vi "ValueAsDouble.vi"(8 "error in (no error)":errorcluster, 11 "Parameter":string="  <value><double>-12.3456</double></value>\n    ") -> (0 "error out":errorcluster, 3 "value":dbl)   [LabVIEW 2009]
doc: "Convert XML-RPC double to LV double"
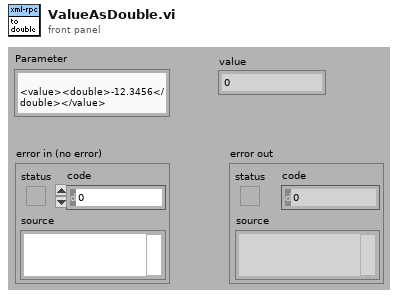
[diagram p1: front panel]
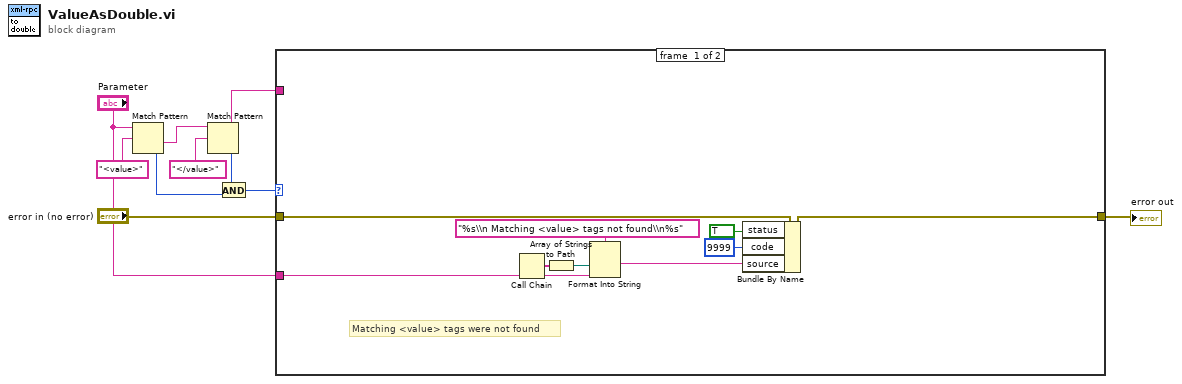
[diagram p0: block diagram]
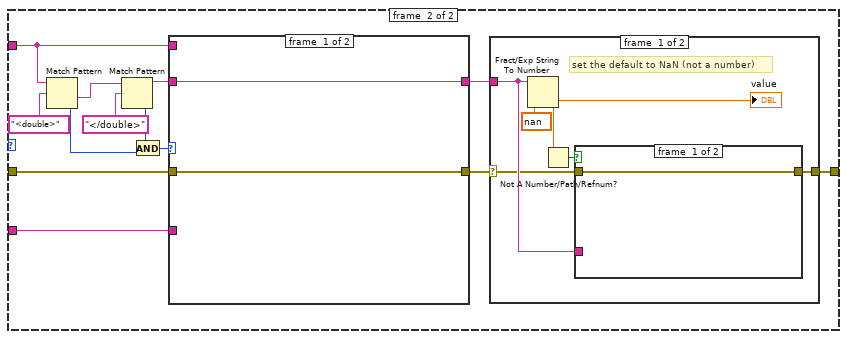
[diagram p2: hidden frame]
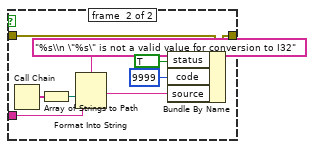
[diagram p3: hidden frame]
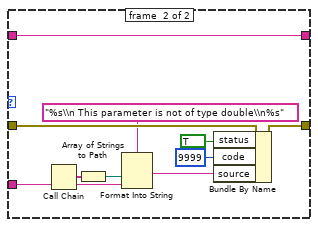
[diagram p5: hidden frame]
diagram:
  n1 = Match Pattern(string="Parameter", regular expression="<value>") -> (after substring=w9:string, offset past match=w2:i32)  [unwired: 1 in, 2 out]
  n2 = Match Pattern(string=w9, regular expression="</value>") -> (before substring=w7:string, offset past match=w3:i32)  [unwired: 1 in, 2 out]
  n3 = And(x=w3, y=w2) -> (x .and. y?=w1:i32)
  n4 = case shown="Default" w1 {
    tunnel: w7 -> [_ w29]
    tunnel: "error in (no error)" -> [w13 w27]
    tunnel: [w12 w22] -> w5
    tunnel: "Parameter" -> [w16 w26]
    frame #0 {
      # "Matching <value> tags were not found"
      n5 = Call Chain() -> (call chain=w19:string[])
      n6 = Array of Strings to Path(0:w19) -> (2:w18:path)  [unwired: 1 in]
      n7 = Format Into String(format string="%s\\n Matching <value> tags not found\\n%s", w18, w16) -> (resulting string=w11:string)  [unwired: 2 in, 1 out]
      n8 = Bundle By Name(cluster=w13, "status"=TRUE, "code"=9999, "source"=w11) -> (w12:errorcluster)
    }
    frame #1 {
      n9 = Match Pattern(string=w29, regular expression="<double>") -> (after substring=w31:string, offset past match=w24:i32)  [unwired: 1 in, 2 out]
      n10 = Match Pattern(string=w31, regular expression="</double>") -> (before substring=w28:string, offset past match=w25:i32)  [unwired: 1 in, 2 out]
      n11 = And(x=w25, y=w24) -> (x .and. y?=w23:i32)
      n12 = case shown="-1" w23 {
        tunnel: w29 -> [_ _]
        tunnel: w28 -> [w51 w52]
        tunnel: [w51 w52] -> w21
        tunnel: w27 -> [w50 w61]
        tunnel: [w50 w60] -> w20
        tunnel: w26 -> [_ w59]
        frame #0 {
        }
        frame #1 {
          n13 = Call Chain() -> (call chain=w58:string[])
          n14 = Array of Strings to Path(0:w58) -> (2:w55:path)  [unwired: 1 in]
          n15 = Format Into String(format string="%s\\n This parameter is not of type double\\n%s", w55, w59) -> (resulting string=w54:string)  [unwired: 2 in, 1 out]
          n16 = Bundle By Name(cluster=w61, "status"=TRUE, "code"=9999, "source"=w54) -> (w60:errorcluster)
        }
      }
      n17 = case shown="No Error" w20 {
        selector: w20 -> [w33 w49]
        tunnel: [w38 w49] -> w22
        tunnel: w21 -> [w37 _]
        frame #0 {
          # "set the default to NaN (not a number)"
          n18 = Fract/Exp String To Number(string=w37, default (0 dbl)=nan ("default (0 DBL)")) -> (number=w35:dbl)  [unwired: 2 in, 1 out]
          "value" <- w35
          n19 = Not A Number/Path/Refnum?(number/path/refnum=w35) -> (NaN/Path/Refnum?=w34:bool)
          n20 = case shown="True" w34 {
            tunnel: w33 -> [w39 w43]
            tunnel: [w39 w42] -> w38
            tunnel: w37 -> [_ w41]
            frame #0 {
            }
            frame #1 {
              n21 = Call Chain() -> (call chain=w44:string[])
              n22 = Array of Strings to Path(0:w44) -> (2:w47:path)  [unwired: 1 in]
              n23 = Format Into String(format string="%s\\n \"%s\" is not a valid value for conversion to I32", w47, w41) -> (resulting string=w48:string)  [unwired: 2 in, 1 out]
              n24 = Bundle By Name(cluster=w43, "status"=TRUE, "code"=9999, "source"=w48) -> (w42:errorcluster)
            }
          }
        }
        frame #1 {
          # "don't try to convert if we can't find a valid tag"
        }
      }
    }
  }
  "error out" <- w5
